vi "testReset.vi"() -> ()   [LabVIEW 2019, in "CodeCoverageTest.lvlib"]
uses:
  CodeCoverageTest.lvlib
  CodeCoverage/CodeCoverage.lvclass/CodeCoverage.ctl
  0ce8ad6e-ca75-4a7e-9425-ba5293e30e67.vi
  Constraint/IsEqual/IsEqual.lvclass
  CodeCoverage/CodeCoverage.lvclass
  Support/Support.lvlib
panel:
  out "error out":errorcluster
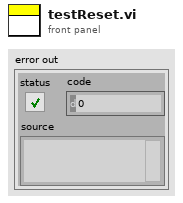
[diagram p1: front panel]
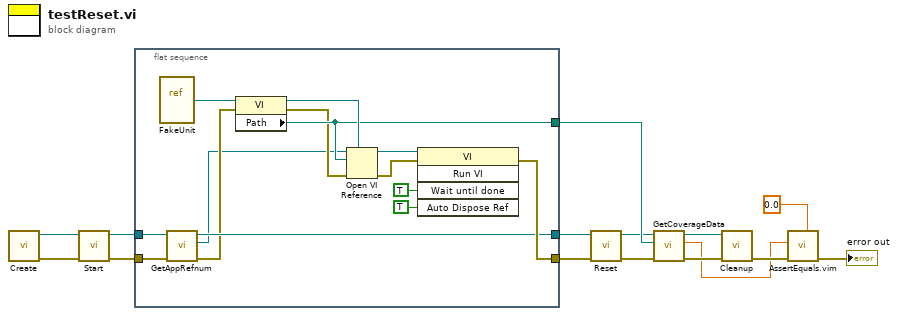
[diagram p0: block diagram]
diagram:
  n1 = call "Create.vi"() -> ("error out"=w14:errorcluster, "CodeCoverage out"=w15:refnum<class "CodeCoverage.lvclass">)  [unwired: 10 in]
  n2 = call "Start.vi"("error in (no error)"=w14, "CodeCoverage in"=w15) -> ("error out"=w10:errorcluster, "CodeCoverage out"=w11:refnum<class "CodeCoverage.lvclass">)  [unwired: 8 in]
  n3 = flat-sequence {
    tunnel: [w19] -> w2
    tunnel: w11 -> [w20]
    tunnel: w10 -> [w18]
    tunnel: [w23] -> w9
    tunnel: [w27] -> w4
    frame #0 {
      n4 = vi-ref "FakeUnit.vi"() -> (w28:refnum<vi>)
      n5 = call "GetAppRefnum.vi"("error in (no error)"=w18, "CodeCoverage in"=w20) -> ("error out"=w17:errorcluster, "App Refnum"=w16:refnum<vi>, "CodeCoverage out"=w19:refnum<class "CodeCoverage.lvclass">)  [unwired: 7 in]
      n6 = property class="VI"(reference=w28, error in=w17) -> (reference out=w29:refnum<vi>, error out=w26:errorcluster, "Path"=w27:path)
      n7 = Open VI Reference(type specifier VI Refnum (for type only)=w29, application reference (local)=w16, vi path=w27, error in (no error)=w26) -> (vi reference=w25:refnum<vi>, error out=w24:errorcluster)  [unwired: 2 in]
      n8 = invoke class="VI" method="Run VI"(reference=w25, error in=w24, "Wait until done"=TRUE ("Wait Until Done"), "Auto Dispose Ref"=TRUE ("Auto Dispose Reference")) -> (error out=w23:errorcluster)  [unwired: 1 in, 4 out]
    }
  }
  n9 = call "Reset.vi"("error in (no error)"=w9, "CodeCoverage in"=w2) -> ("error out"=w3:errorcluster, "CodeCoverage out"=w1:refnum<class "CodeCoverage.lvclass">)  [unwired: 8 in]
  n10 = call "GetCoverageData.vi"("error in (no error)"=w3, "VI Path"=w4, "CodeCoverage in"=w1) -> ("error out"=w12:errorcluster, "Coverage Percentage"=w7:dbl, "CodeCoverage out"=w13:refnum<class "CodeCoverage.lvclass">)  [unwired: 6 in]
  n11 = call "Cleanup.vi"("error in (no error)"=w12, "CodeCoverage in"=w13) -> ("error out"=w8:errorcluster)  [unwired: 9 in]
  n12 = call "AssertEquals.vim"("Expected"=0.0 ("Coverage Percentage"), "error in (no error)"=w8, "Actual"=w7) -> ("error out"=→"error out":errorcluster)  [unwired: 8 in]
